vi "Keithley 27XX Temperature (Thermocouple).vi"() -> ()   [LabVIEW 2020]
doc: "This example VI shows how to use thermocouples to take a temperature measurement.\n\nNote:\nFor front panel measurements, make sure the Input switch is in the out position(F)\nFor plug-in card measurements, make sure the Input switch is in the in poisition(R)"
uses:
  <instrlib>/Keithley 27XX/Public/Configure/Measurement Specific/Configure Thermocouple.vi
  <instrlib>/Keithley 27XX/Public/Data/Read Single Point.vi
  <instrlib>/Keithley 27XX/Keithley 27XX.lvlib
panel:
  in  "Serial Configuration":T1={"Baud Rate (9600)"=9600, "Flow Control (1: XON/XOFF)"=1, "Termination Char (0:CR)"=0} {"Termination Char (0:CR)" items=["CR", "LF", "CRLF (Do not use)", "LFCR (Do not use)"]; "Flow Control (1: XON/XOFF)" items=["None", "XON/XOFF", "RTS/CTS (2701 Only)", "XON/XOFF & RTS/CTS (2701 Only)"]; "Baud Rate (9600)" items=["300"=300, "600"=600, "1200"=1200, "2400"=2400, "4800"=4800, "9600"=9600, "19.2k"=19200, "38.4k (2701 Only)"=38400, "57.6k (2701 Only)"=57600, "115.2k (2701 Only)"=115200]}
  in  "Channel (101)":string="101"
  in  "Temperature (0: Celsius)":u16(ring) items=["Celsius", "Fahrenheit", "Kelvin"]
  in  "Simulated Refence Temperature (23)":dbl=23.0
  in  "Reference Junction Type (0: Simulated)":u16(ring) items=["Simulated", "Internal", "External"]
  in  "Thermocouple Type (1: K)":u16(ring)=1 items=["J", "K", "T", "E", "R", "S", "B", "N"]
  in  "VISA resource name":refnum<visa-resource-name>
  out "Measurement Data":dbl
  # "*For front panel measurements, make sure the Input switch is in the out position(F)*\n  For plug-in card measurements, make sure the Input switch is in the in position(R)"
  # "© 2005 National Instruments Corporation.  ALL RIGHTS RESERVED."
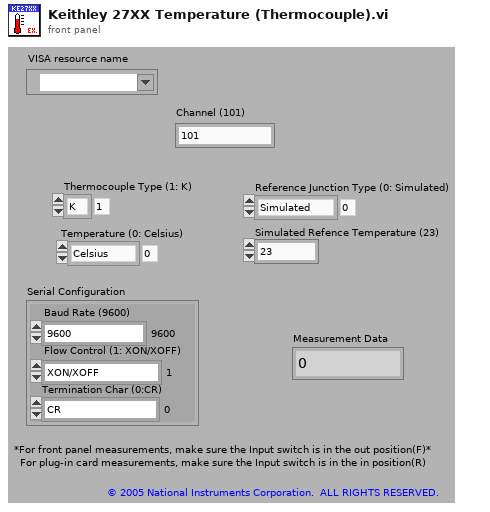
[diagram p1: front panel]
types:
  T1 = cluster{"Baud Rate (9600)":u32, "Flow Control (1: XON/XOFF)":u16, "Termination Char (0:CR)":u16}
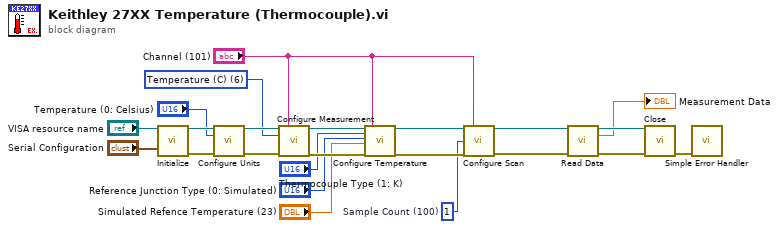
[diagram p0: block diagram]
diagram:
  w3 = 1  # Sample Count (100)
  w21 = u16 6 items=["DC Voltage", "AC Voltage", "DC Current", "AC Current", "Resistance", "Four-Wire Resistance", "Temperature (C)", "Frequency", "Period", "Continuity"] ("Function (0: DC Voltage)")
  n1 = call <instrlib>:"Initialize.vi"("VISA resource name"="VISA resource name", "Serial Configuration"="Serial Configuration") -> ("VISA resource name out"=w20:refnum<visa-resource-name>, "error out"=w6:errorcluster)  [unwired: 12 in]
  n2 = call <instrlib>:"Configure Units.vi"("VISA resource name"=w20, "Temperature (0: Celsius)"="Temperature (0: Celsius)", "error in (no error)"=w6) -> ("VISA resource name out"=w22:refnum<visa-resource-name>, "error out"=w5:errorcluster)  [unwired: 11 in]
  n3 = call <instrlib>:"Configure Measurement.vi"("VISA resource name"=w22, "Scan List (Empty)"="Channel (101)", "Function (0: DC Voltage)"=w21, "error in (no error)"=w5) -> ("VISA resource name out"=w4:refnum<visa-resource-name>, "error out"=w23:errorcluster)  [unwired: 10 in]
  n4 = call-poly <instrlib>:"Configure Temperature.vi"("VISA resource name"=w4, "Thermocouple Type (1: K)"="Thermocouple Type (1: K)", "Reference Junction Type (0: Simulated)"="Reference Junction Type (0: Simulated)", "Simulated Reference Temperature (23 deg C)"="Simulated Refence Temperature (23)", "error in (no error)"=w23, "Scan List (Empty)"="Channel (101)") -> ("VISA resource name out"=w13:refnum<visa-resource-name>, "error out"=w12:errorcluster)  [unwired: 12 in]
  n5 = call <instrlib>:"Configure Scan.vi"("VISA resource name"=w13, "Channel List (101:110)"="Channel (101)", "Sample Count (100)"=w3, "error in (no error)"=w12) -> ("VISA resource name out"=w10:refnum<visa-resource-name>, "error out"=w11:errorcluster)  [unwired: 10 in]
  n6 = call-poly <instrlib>:"Read Data.vi"("VISA resource name"=w10, "error in (no error)"=w11) -> ("VISA resource name out"=w7:refnum<visa-resource-name>, "Measurement Data"=→"Measurement Data":dbl, "error out"=w8:errorcluster)  [unwired: 11 in]
  n7 = call <instrlib>:"Close.vi"("VISA resource name"=w7, "error in (no error)"=w8) -> ("error out"=w15:errorcluster)  [unwired: 13 in]
  n8 = call <vilib>:"Simple Error Handler.vi"("error in (no error)"=w15) -> ()  [unwired: 4 in, 5 out]
